vi "Motor.vi"(0 "Enum":enum16{"Start", "Run", "End"}(ring), 1 "Motor":dbl) -> ()   [LabVIEW 2012]
uses:
  TypeDefs/PWM Module 1.ctl
  <vilib>/Rock Robotics/SystemInterfaces/Typedef/FPGA_TypedefDigitalModule.ctl
  <vilib>/Rock Robotics/SystemInterfaces/DIO/FPGA_DIOPWMChannel.ctl
  <vilib>/Rock Robotics/SystemInterfaces/DIO/FPGA_DIORelayChannel.ctl
  <vilib>/Rock Robotics/WPI/MotorControl/WPI_MotorControlOpen Jaguar.vi
panel:
  in  "PWM Module (DIO A)":T1={"Module"=enum."Digital Module 1", "Unassigned"=enum."PWM 1", "Unassigned"=enum."PWM 2", "Unassigned"=enum."PWM 3", "Unassigned"=enum."PWM 4", "Unassigned"=enum."PWM 5", "Unassigned"=enum."PWM 6", "Unassigned"=enum."PWM 7", "Unassigned"=enum."PWM 8", "Unassigned"=enum."PWM 9", "Unassigned"=enum."PWM 10", "Unassigned"=enum."Relay 1", "Unassigned"=enum."Relay 2", "Unassigned"=enum."Relay 3", "Unassigned"=enum."Relay 4", "Unassigned"=enum."Relay 5", "Unassigned"=enum."Relay 6", "Unassigned"=enum."Relay 7", "Unassigned "=enum."Relay 8"}
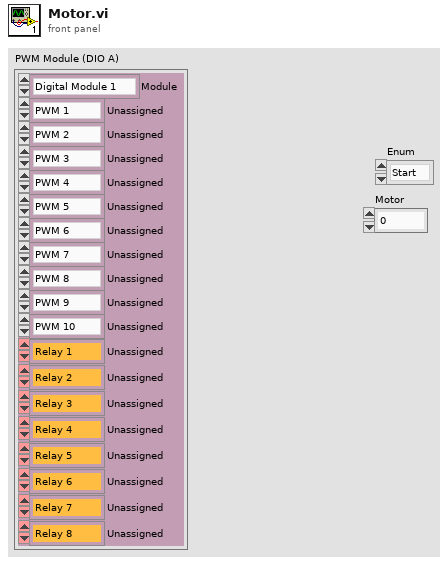
[diagram p1: front panel]
types:
  T1 = typedef "PWM Module 1.ctl" = cluster{"Module":T2, "Unassigned":T3, "Unassigned":T3, "Unassigned":T3, "Unassigned":T3, "Unassigned":T3, "Unassigned":T3, "Unassigned":T3, "Unassigned":T3, "Unassigned":T3, "Unassigned":T3, "Unassigned":T4, "Unassigned":T4, "Unassigned":T4, "Unassigned":T4, "Unassigned":T4, "Unassigned":T4, "Unassigned":T4, "Unassigned ":T4}
  T2 = typedef "FPGA_TypedefDigitalModule.ctl" = enum16{"Digital Module 1", "Digital Module 2"}
  T3 = typedef "FPGA_DIOPWMChannel.ctl" = enum8{"PWM 1", "PWM 2", "PWM 3", "PWM 4", "PWM 5", "PWM 6", "PWM 7", "PWM 8", "PWM 9", "PWM 10", "Invalid"}
  T4 = typedef "FPGA_DIORelayChannel.ctl" = enum8{"Relay 1", "Relay 2", "Relay 3", "Relay 4", "Relay 5", "Relay 6", "Relay 7", "Relay 8", "Invalid"}
  T5 = typedef "WPI_MotorControlDeviceRef.ctl" = cluster{"DeviceStatus":errorcluster, "Type":enum16{"PWM", "CAN"}, "PWM":cluster{"Digital Module":T2, "PWM Channel":T3, "DeadBand":T6}, "CAN":cluster{"Device Number":u8, "Control Mode":T7, "Semaphore":T8, "Max Vout":dbl}, "Invert":bool, "TransformRef":T9, "InvTransformRef":T9}
  T6 = typedef "WPI_PWMDeadband.ctl" = cluster{"Name":string, "maxPositivePwm":i32, "minPositivePwm":i32, "centerPwm":i32, "maxNegativePwm":i32, "minNegativePwm":i32, "angularRange":u16}
  T7 = typedef "WPI_CANJaguar_ControlMode.ctl" = enum8{"Percent VBus", "Current", "Speed", "Position", "Voltage"}
  T8 = typedef "Semaphore RefNum" = refnum<k1>
  T9 = typedef "WPI_PWMTransform_ConPane.ctl" = refnum<vi>
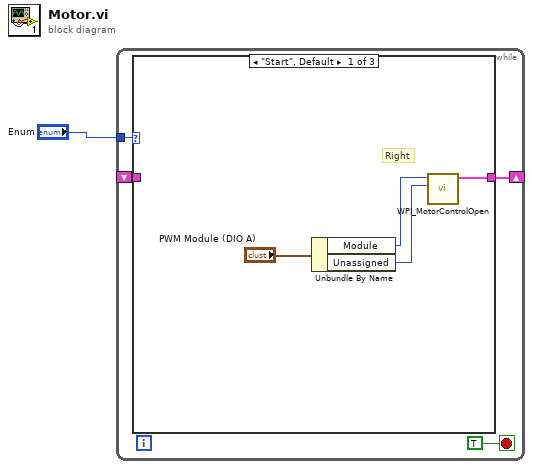
[diagram p0: block diagram]
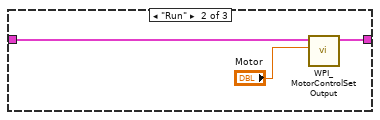
[diagram p2: hidden frame]
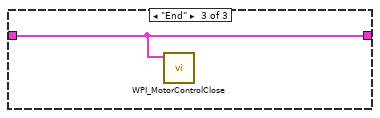
[diagram p3: hidden frame]
diagram:
  n1 = while {
    shift-right: [w4] -> _
    shift-left: _ -> [w3]
    tunnel: "Enum" -> [w2]
    stop <- TRUE stop-if-true
    n2 = case shown="\"Start\", Default" w2 {
      tunnel: [w9 w11 w13] -> w4
      tunnel: w3 -> [_ w12 w13]
      frame "Start", Default {
        # "Right"
        n3 = Unbundle By Name("PWM Module (DIO A)") -> ("Module"=w7:T2, "Unassigned"=w8:T3)
        n4 = call-poly <vilib>:"WPI_MotorControlOpen.vi"("PWM Channel"=w8, "Digital Module (Module 1)"=w7) -> ("MotorControlDeviceRef"=w9:T5)  [unwired: 8 in, 1 out]
      }
      frame "Run" {
        n5 = call <vilib>:"WPI_MotorControlSetOutput.vi"("Output"="Motor", "MotorControlDevRef"=w12) -> ("MotorControlDevRef"=w11:T5)  [unwired: 7 in, 2 out]
      }
      frame "End" {
        n6 = call <vilib>:"WPI_MotorControlClose.vi"("MotorControlDevRef"=w13) -> ()  [unwired: 10 in, 1 out]
      }
    }
  }
